vi "GetParam.vi"(8 "error in (no error)":errorcluster caption="entrée d'erreur (pas d'erreur)", 11 "Sigmoid_kernel.lvclass":refnum<class "Sigmoid_kernel.lvclass">) -> (0 "error out":errorcluster caption="sortie d'erreur", 2 "sigmoid_kernel":cluster{"gamma":string, "coef0":dbl}={"gamma"="None", "coef0"=1.0}, 3 "Sigmoid_kernel.lvclass":refnum<class "Sigmoid_kernel.lvclass">)   [LabVIEW 2020, in "Sigmoid_kernel.lvclass"]
doc: "Get Parameters"
uses:
  Sigmoid_kernel.lvclass
  Sigmoid_kernel.lvclass/Sigmoid_kernel.ctl
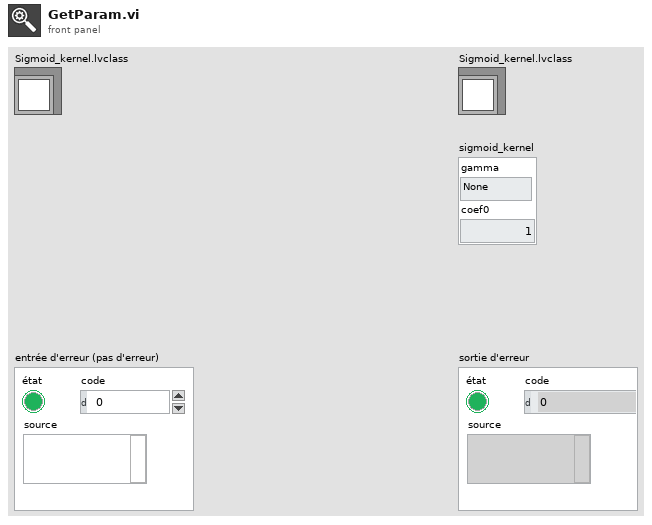
[diagram p1: front panel]
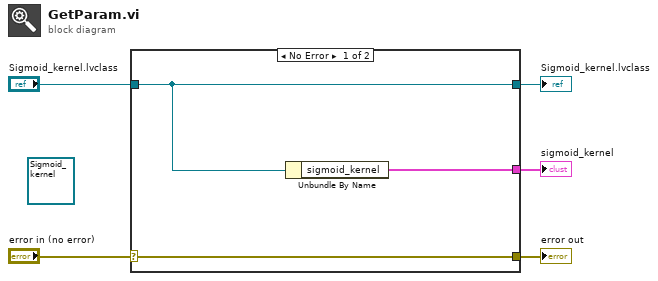
[diagram p0: block diagram]
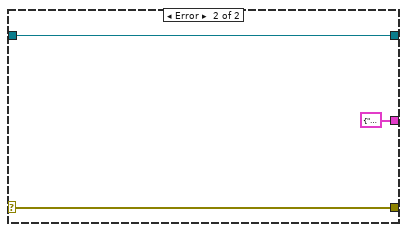
[diagram p2: hidden frame]
diagram:
  (unwired) refnum<class "Sigmoid_kernel.lvclass"> refnum ("Sigmoid_kernel.lvclass")
  n1 = case shown="No Error" "error in (no error)" {
    selector: "error in (no error)" -> [w8 w10]
    tunnel: [w8 w10] -> w4
    tunnel: [w7 w11] -> w2
    tunnel: "Sigmoid_kernel.lvclass" -> [w7 w11]
    tunnel: [w6 cluster{"gamma":string, "coef0":dbl} {"gamma"="", "coef0"=0.0} ("sigmoid_kernel")] -> w1
    frame No Error {
      n2 = Unbundle By Name(w7) -> ("sigmoid_kernel"=w6:cluster{"gamma":string, "coef0":dbl})
    }
    frame Error {
    }
  }
  "error out" <- w4
  "Sigmoid_kernel.lvclass" <- w2
  "sigmoid_kernel" <- w1
